vi "Determine Stage Transition Index.vi"(7 "Stage Dwell Limit":u16, 10 "Previous Inj Event Boolean State Data":T1, 11 "Inj Event Boolean State Data":T1) -> (0 "Trigger":u32, 1 "New Event Written to FIFO?":bool, 2 "New Stage Transition Index":u32, 3 "Inj Event Boolean State Data out":T1)   [LabVIEW 2015]
uses:
  Types/Injection Capture Core Boolean State Data.ctl
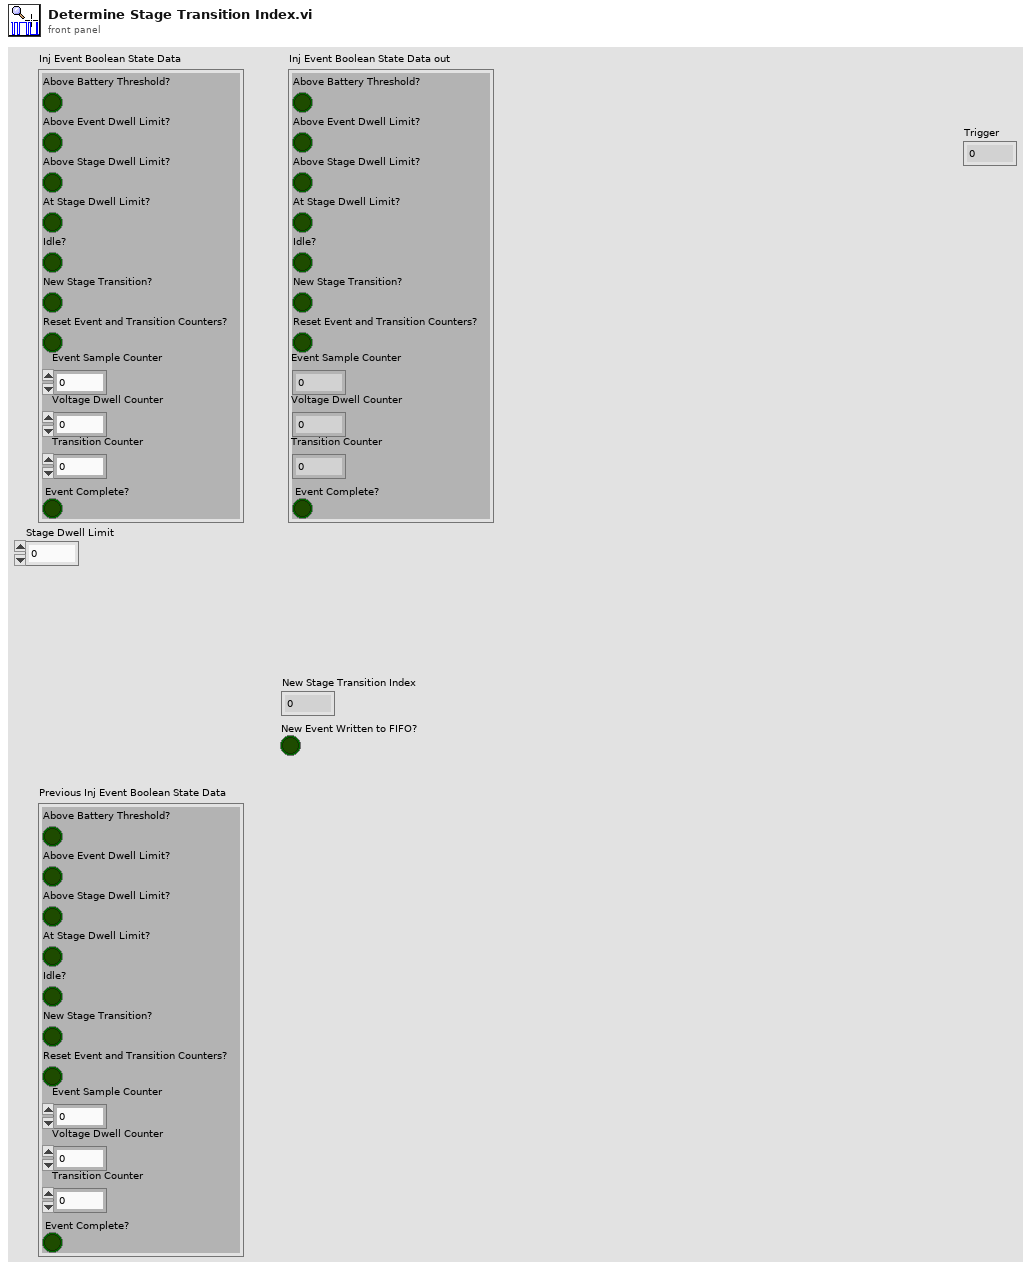
[diagram p1: front panel]
types:
  T1 = typedef "Injection Capture Core Boolean State Data.ctl" = cluster{"Above Battery Threshold?":bool, "Above Event Dwell Limit?":bool, "Above Stage Dwell Limit?":bool, "At Stage Dwell Limit?":bool, "Idle?":bool, "New Stage Transition?":bool, "Reset Event and Transition Counters?":bool, "Event Sample Counter":u16, "Voltage Dwell Counter":u32, "Transition Counter":u8, "Event Complete?":bool}
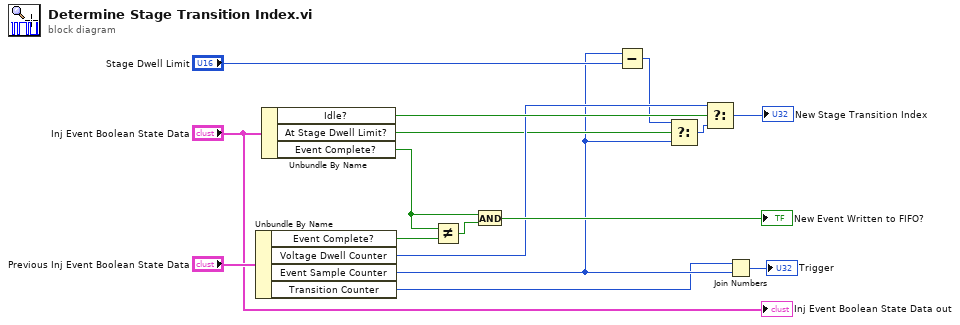
[diagram p0: block diagram]
diagram:
  n1 = Unbundle By Name("Previous Inj Event Boolean State Data") -> ("Event Complete?"=w14:bool, "Voltage Dwell Counter"=w9:u32, "Event Sample Counter"=w3:u16, "Transition Counter"=w2:u8)
  n2 = Unbundle By Name("Inj Event Boolean State Data") -> ("Idle?"=w10:bool, "At Stage Dwell Limit?"=w7:bool, "Event Complete?"=w8:bool)
  n3 = Not Equal?(x=w8, y=w14) -> (x != y?=w15:bool)
  n4 = And(x=w8, y=w15) -> (x .and. y?=→"New Event Written to FIFO?":bool)
  n5 = Subtract(x=w3, y="Stage Dwell Limit") -> (x-y=w5:u16)
  n6 = Select(t=w5, s=w7, f=w3) -> (s? t:f=w6:u16)
  n7 = Select(t=w9, s=w10, f=w6) -> (s? t:f=→"New Stage Transition Index":u32)
  n8 = Join Numbers(hi=w2, lo=w3) -> ((hi.lo)=→"Trigger":u32)
  "Inj Event Boolean State Data out" <- "Inj Event Boolean State Data"
